vi "get_counts.vi"(8 "error in":errorcluster, 11 "Detection length (ms)":dbl=20.0 min=1.0) -> (0 "error out":errorcluster, 3 "Counts":u32=198)   [LabVIEW 2012]
uses:
  <vilib>/DAQmx/read.llb/DAQmx Read (Counter 1D U32 1Chan NSamp).vi
  <vilib>/DAQmx/create/channels.llb/DAQmx Create Channel (CI-Count Edges).vi
  <vilib>/DAQmx/configure/timing.llb/DAQmx Timing (Sample Clock).vi
  <vilib>/DAQmx/miscellaneous.llb/DAQmx Fill In Error Info.vi
  <resource>/objmgr/daqmx.rc
panel:
  out "data":u32[](graph)=[0, 0, 1, 0, 1, 0, 2, 0, 2, 4, 2, 2, 0, 2, 0, 0, 2, 1, 2, 1]
  out "Output":bool=TRUE
  in  "Threshold":dbl=200.0
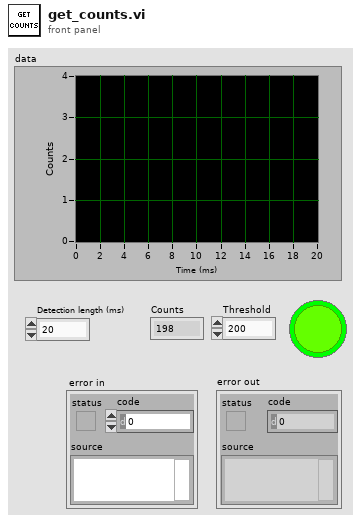
[diagram p1: front panel]
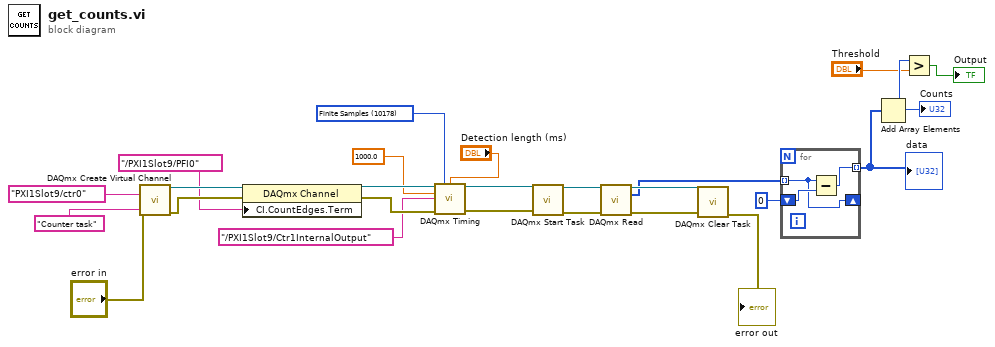
[diagram p0: block diagram]
diagram:
  w20 = 10178 items=["Finite Samples"=10178, "Continuous Samples"=10123, "Hardware Timed Single Point"=12522] ("sample mode")
  n1 = call-poly <vilib>:"DAQmx Create Virtual Channel.vi"("counter"=tag "PXI1Slot9/ctr0", "name to assign"="Counter task", "error in"="error in") -> ("task out"=w24:refnum<k21>, "error out"=w23:errorcluster)  [unwired: 11 in]
  n2 = property class="DAQmx Channel"(reference=w24, error in=w23, "CI.CountEdges.Term"=tag "/PXI1Slot9/PFI0") -> (reference out=w21:refnum<k21>, error out=w19:errorcluster)
  n3 = call-poly <vilib>:"DAQmx Timing.vi"("task/channels in"=w21, "sample mode"=w20, "samples per channel"="Detection length (ms)", "rate"=1000.0, "source"=tag "/PXI1Slot9/Ctr1InternalOutput", "error in"=w19) -> ("task out"=w5:refnum<k21>, "error out"=w4:errorcluster)  [unwired: 8 in]
  n4 = call <vilib>:"DAQmx Start Task.vi"("task/channels in"=w5, "error in"=w4) -> ("task out"=w9:refnum<k21>, "error out"=w10:errorcluster)  [unwired: 12 in]
  n5 = call-poly <vilib>:"DAQmx Read.vi"("task/channels in"=w9, "error in"=w10) -> ("task out"=w15:refnum<k21>, "data"=w8:u32[], "error out"=w14:errorcluster)  [unwired: 11 in]
  n6 = call <vilib>:"DAQmx Clear Task.vi"("task in"=w15, "error in"=w14) -> ("error out"=→"error out":errorcluster)  [unwired: 13 in]
  n7 = for {
    tunnel: w8 -> [w26] mode=indexing
    tunnel: [w27] -> w6 mode=indexing
    shift-right: [w26] -> _
    shift-left: u32 0 ("Numeric") -> [w28]
    n8 = Subtract(x=w26, y=w28) -> (x-y=w27:u32)
  }
  "data" <- w6
  n9 = Add Array Elements(numeric array=w6) -> (sum=w13:u32)
  "Counts" <- w13
  n10 = Greater?(x=w13, y="Threshold") -> (0:→"Output":bool)
